vi "LookUpTableCreator.vi"() -> ()   [LabVIEW 2016]
uses:
  Common_SubVI/cRIO Convert Thermocouple Readings.llb/Thermocouple Type.ctl
panel:
  out "Thermocouple Voltage":sgl format="%0.6f"
  out "Test Value":sgl
  out "Lookup Table":sgl[](array[numeric])
  out "Resolution":dbl
  in  "Number of Values":i32=100
  in  "End Value":dbl=0.0782
  in  "Start Value":dbl
  # "This is the value the lookup\ntable algorithm will return given the\ntest value reading of 0.003"
  # "This is the actual value Test Value\nshould have found"
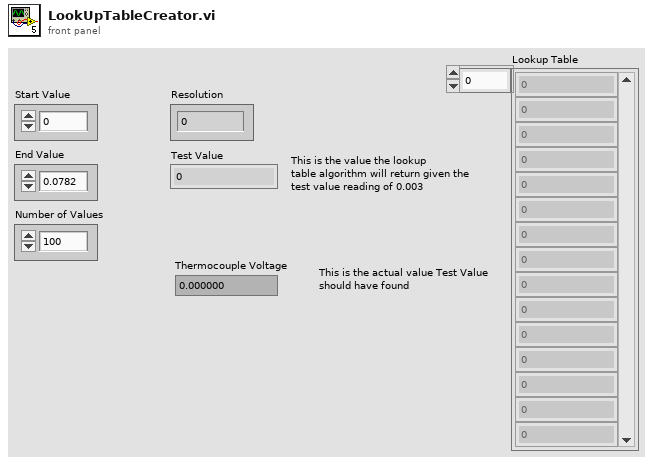
[diagram p1: front panel]
types:
  T1 = typedef "Thermocouple Type.ctl" = u16
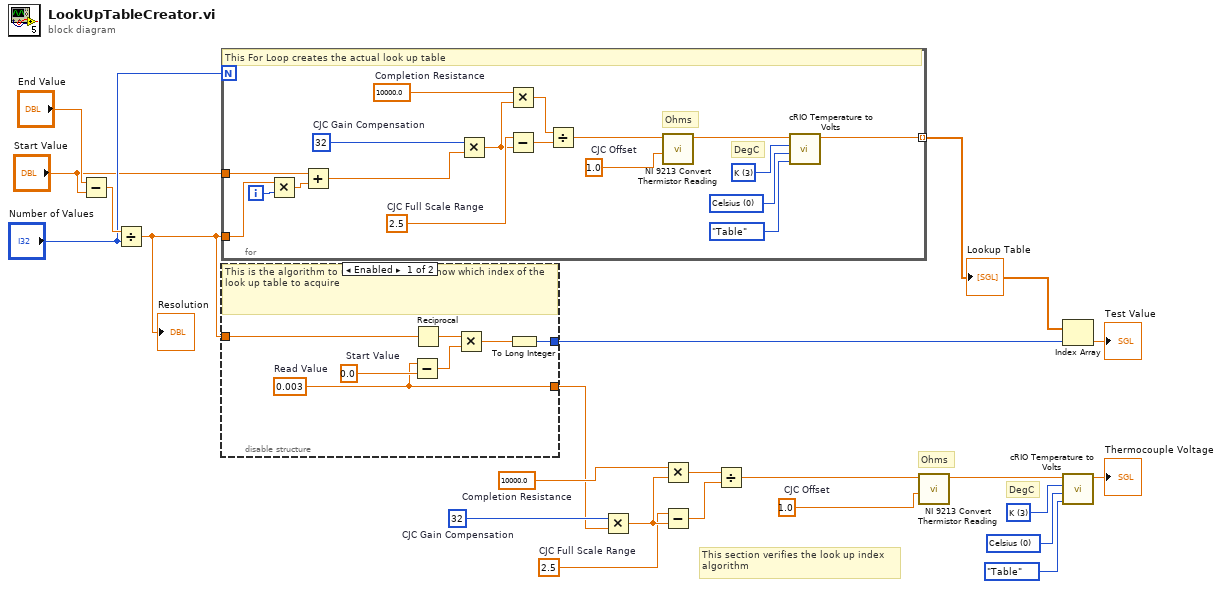
[diagram p0: block diagram]
diagram:
  w4 = u16 0 items=["Celsius", "Fahrenheit", "Kelvin", "Rankine"] ("Temperature Units")
  w5 = T1 3 items=["B", "E", "J", "K", "R", "S", "T", "N"] ("ThermocoupleType")
  w14 = 1.0  # CJC Offset
  w10 = sgl 2.5  # CJC Full Scale Range
  w7 = 32  # CJC Gain Compensation
  w9 = sgl 10000.0  # Completion Resistance
  # "This section verifies the look up index\nalgorithm"
  # "Ohms"
  # "DegC"
  n1 = Subtract(x="End Value", y="Start Value") -> (x-y=w21:dbl)
  n2 = Divide(x=w21, y="Number of Values") -> (x/y=w18:dbl)
  "Resolution" <- w18
  n3 = for {
    N: "Number of Values" -> [_]
    tunnel: "Start Value" -> [w25]
    tunnel: [w23] -> w17 mode=indexing
    tunnel: w18 -> [w27]
    i -> [w28]
    w39 = u16 0 items=["Celsius", "Fahrenheit", "Kelvin", "Rankine"] ("Temperature Units")
    w38 = T1 3 items=["B", "E", "J", "K", "R", "S", "T", "N"] ("ThermocoupleType")
    w29 = 1.0  # CJC Offset
    w33 = sgl 2.5  # CJC Full Scale Range
    w36 = 32  # CJC Gain Compensation
    w34 = sgl 10000.0  # Completion Resistance
    # "Ohms"
    # "DegC"
    # "This For Loop creates the actual look up table"
    n4 = Multiply(x=w27, y=w28) -> (x*y=w26:dbl)
    n5 = Add(x=w25, y=w26) -> (x+y=w24:dbl)
    n6 = Multiply(x=w36, y=w24) -> (x*y=w32:dbl)
    n7 = Multiply(x=w34, y=w32) -> (x*y=w30:dbl)
    n8 = Subtract(x=w33, y=w32) -> (x-y=w31:dbl)
    n9 = Divide(x=w30, y=w31) -> (x/y=w35:dbl)
    n10 = call "NI 9213 Convert Thermistor Reading.vi"("CJC Offset"=w29, "Rt"=w35) -> ("CJC Temperature"=w37:sgl)  [unwired: 1 in, 8 out]
    n11 = call "cRIO Temperature to Volts.vi"("Scale Type"=enum16{"Polynomial", "Table"}."Table", "Temperature Units"=w39, "ThermocoupleType"=w38, "Temperature"=w37) -> ("Thermocouple Voltage"=w23:sgl)  [unwired: 3 out]
  }
  "Lookup Table" <- w17
  n12 = disable-structure shown="Enabled" {
    disable-tunnel: w18 -> [w44 _]
    disable-tunnel: [w42 _] -> w16
    disable-tunnel: [w41 _] -> w2
    frame Enabled {
      w41 = 0.003  # Read Value
      w47 = sgl 0.0  # Start Value
      # "This is the algorithm to use in the FPGA to know which index of the look up table to acquire"
      n13 = Subtract(x=w41, y=w47) -> (x-y=w46:dbl)
      n14 = Reciprocal(x=w44) -> (1/x=w45:dbl)
      n15 = Multiply(x=w45, y=w46) -> (x*y=w43:dbl)
      n16 = To Long Integer(number=w43) -> (32bit integer=w42:i32)
    }
    frame Disabled {
    }
  }
  n17 = Multiply(x=w7, y=w2) -> (x*y=w11:dbl)
  n18 = Multiply(x=w9, y=w11) -> (x*y=w13:dbl)
  n19 = Subtract(x=w10, y=w11) -> (x-y=w12:dbl)
  n20 = Divide(x=w13, y=w12) -> (x/y=w8:dbl)
  n21 = call "NI 9213 Convert Thermistor Reading.vi"("CJC Offset"=w14, "Rt"=w8) -> ("CJC Temperature"=w6:sgl)  [unwired: 1 in, 8 out]
  n22 = Index Array(array=w17, index=w16) -> (element=→"Test Value":sgl)
  n23 = call "cRIO Temperature to Volts.vi"("Scale Type"=enum16{"Polynomial", "Table"}."Table", "Temperature Units"=w4, "ThermocoupleType"=w5, "Temperature"=w6) -> ("Thermocouple Voltage"=→"Thermocouple Voltage":sgl)  [unwired: 3 out]
